vi "ParamByteArray.vi"(2 "idx":u8, 3 "Param Nm":u8) -> (5 "Byte3":u8, 6 "Byte2":u8, 7 "Byte1":u8, 8 "Byte0":u8)   [LabVIEW 2017]
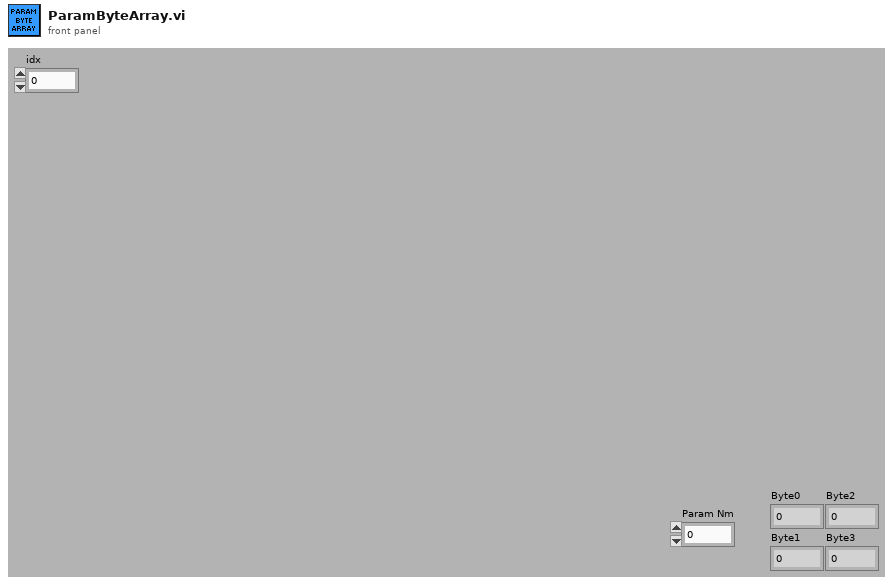
[diagram p1: front panel]
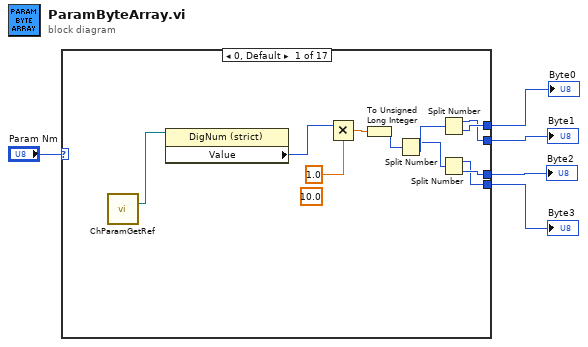
[diagram p0: block diagram]
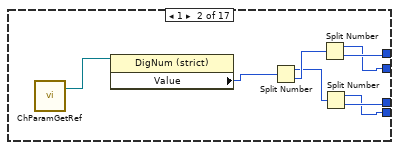
[diagram p2: hidden frame]
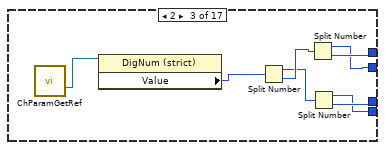
[diagram p3: hidden frame]
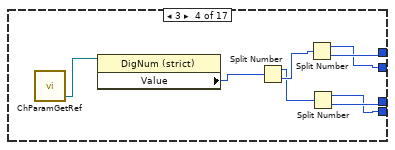
[diagram p4: hidden frame]
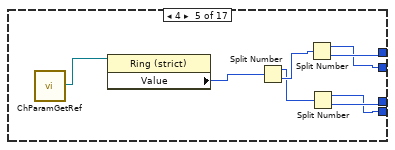
[diagram p5: hidden frame]
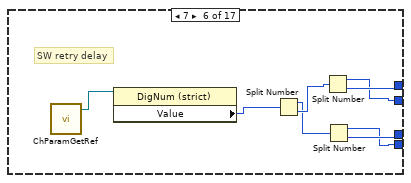
[diagram p6: hidden frame]
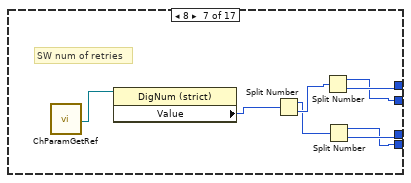
[diagram p7: hidden frame]
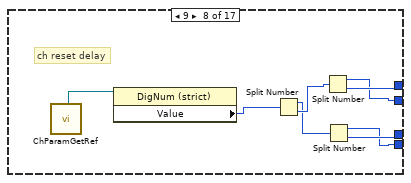
[diagram p8: hidden frame]
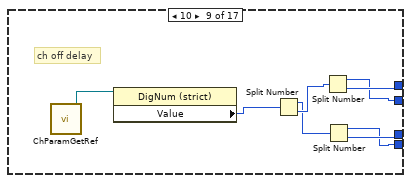
[diagram p9: hidden frame]
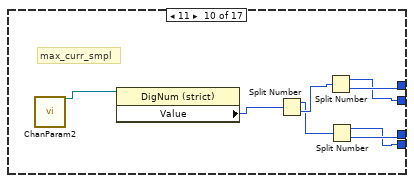
[diagram p10: hidden frame]
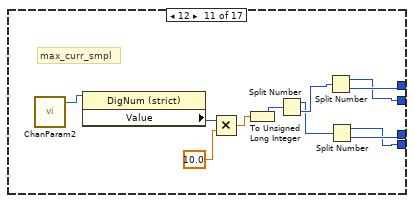
[diagram p11: hidden frame]
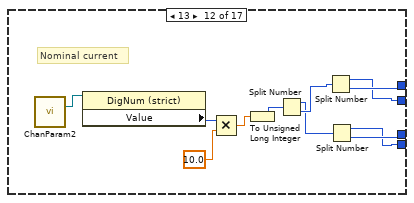
[diagram p12: hidden frame]
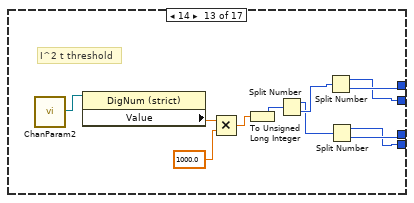
[diagram p13: hidden frame]
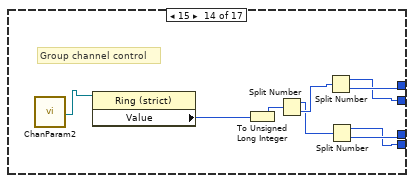
[diagram p14: hidden frame]
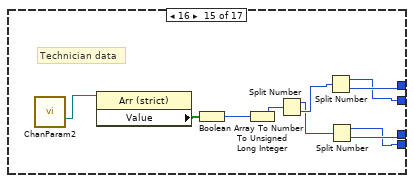
[diagram p15: hidden frame]
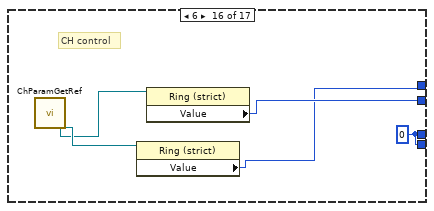
[diagram p16: hidden frame]
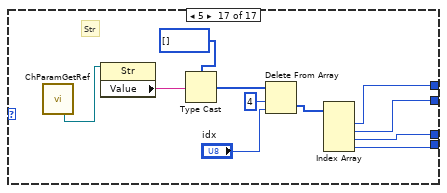
[diagram p17: hidden frame]
diagram:
  n1 = case shown="0, Default" "Param Nm" {
    tunnel: [w14 w20 w28 w36 w45 w53 w61 w69 w77 w85 w97 w108 w119 w128 w138 w142 w150] -> w4
    tunnel: [w13 w19 w27 w35 w44 w52 w60 w68 w76 w84 w96 w107 w118 w127 w137 w143 w149] -> w3
    tunnel: [w12 w18 w26 w34 w43 w51 w59 w67 w75 w83 w95 w106 w117 w126 w136 w141 w148] -> w2
    tunnel: [w11 w17 w25 w33 w42 w50 w58 w66 w74 w82 w94 w105 w116 w125 w135 w141 w147] -> w1
    frame 0, Default {
      (unwired) 10.0 ("y")
      n2 = call "ChParamGetRef.vi"() -> ("Current Threshold  out"=w6:refnum<vi>)  [unwired: 15 in, 12 out]
      n3 = property class="DigNum (strict)"(reference=w6) -> ("Value"=w7:u32)  [unwired: 1 in, 2 out]
      n4 = Multiply(x=w7, y=1.0) -> (x*y=w10:dbl)
      n5 = To Unsigned Long Integer(number=w10) -> (unsigned 32bit integer=w9:u32)
      n6 = Split Number(x=w9) -> (hi(x)=w15:u16, lo(x)=w16:u16)
      n7 = Split Number(x=w16) -> (hi(x)=w13:u8, lo(x)=w14:u8)
      n8 = Split Number(x=w15) -> (hi(x)=w11:u8, lo(x)=w12:u8)
    }
    frame 1 {
      n9 = call "ChParamGetRef.vi"() -> ("Channel On Delay out"=w23:refnum<vi>)  [unwired: 15 in, 12 out]
      n10 = property class="DigNum (strict)"(reference=w23) -> ("Value"=w24:u32)  [unwired: 1 in, 2 out]
      n11 = Split Number(x=w24) -> (hi(x)=w21:u16, lo(x)=w22:u16)
      n12 = Split Number(x=w22) -> (hi(x)=w19:u8, lo(x)=w20:u8)
      n13 = Split Number(x=w21) -> (hi(x)=w17:u8, lo(x)=w18:u8)
    }
    frame 2 {
      n14 = call "ChParamGetRef.vi"() -> ("Retry Delay out"=w31:refnum<vi>)  [unwired: 15 in, 12 out]
      n15 = property class="DigNum (strict)"(reference=w31) -> ("Value"=w32:u32)  [unwired: 1 in, 2 out]
      n16 = Split Number(x=w32) -> (hi(x)=w29:u16, lo(x)=w30:u16)
      n17 = Split Number(x=w30) -> (hi(x)=w27:u8, lo(x)=w28:u8)
      n18 = Split Number(x=w29) -> (hi(x)=w25:u8, lo(x)=w26:u8)
    }
    frame 3 {
      n19 = call "ChParamGetRef.vi"() -> ("Number Of Retry out"=w39:refnum<vi>)  [unwired: 15 in, 12 out]
      n20 = property class="DigNum (strict)"(reference=w39) -> ("Value"=w40:u32)  [unwired: 1 in, 2 out]
      n21 = Split Number(x=w40) -> (hi(x)=w37:u16, lo(x)=w38:u16)
      n22 = Split Number(x=w38) -> (hi(x)=w35:u8, lo(x)=w36:u8)
      n23 = Split Number(x=w37) -> (hi(x)=w33:u8, lo(x)=w34:u8)
    }
    frame 4 {
      n24 = call "ChParamGetRef.vi"() -> ("Active on startup out"=w41:refnum<vi>)  [unwired: 15 in, 12 out]
      n25 = property class="Ring (strict)"(reference=w41) -> ("Value"=w48:u8)  [unwired: 1 in, 2 out]
      n26 = Split Number(x=w48) -> (hi(x)=w46:u8, lo(x)=w47:u8)
      n27 = Split Number(x=w47) -> (hi(x)=w44:u8, lo(x)=w45:u8)
      n28 = Split Number(x=w46) -> (hi(x)=w42:u8, lo(x)=w43:u8)
    }
    frame 7 {
      # "SW retry delay"
      n29 = call "ChParamGetRef.vi"() -> ("SW Retry Delay out"=w49:refnum<vi>)  [unwired: 15 in, 12 out]
      n30 = property class="DigNum (strict)"(reference=w49) -> ("Value"=w56:u32)  [unwired: 1 in, 2 out]
      n31 = Split Number(x=w56) -> (hi(x)=w54:u16, lo(x)=w55:u16)
      n32 = Split Number(x=w55) -> (hi(x)=w52:u8, lo(x)=w53:u8)
      n33 = Split Number(x=w54) -> (hi(x)=w50:u8, lo(x)=w51:u8)
    }
    frame 8 {
      # "SW num of retries"
      n34 = call "ChParamGetRef.vi"() -> ("SW Number Of Retry out"=w57:refnum<vi>)  [unwired: 15 in, 12 out]
      n35 = property class="DigNum (strict)"(reference=w57) -> ("Value"=w64:u32)  [unwired: 1 in, 2 out]
      n36 = Split Number(x=w64) -> (hi(x)=w62:u16, lo(x)=w63:u16)
      n37 = Split Number(x=w63) -> (hi(x)=w60:u8, lo(x)=w61:u8)
      n38 = Split Number(x=w62) -> (hi(x)=w58:u8, lo(x)=w59:u8)
    }
    frame 9 {
      # "ch reset delay"
      n39 = call "ChParamGetRef.vi"() -> ("Reset Status Delay out"=w65:refnum<vi>)  [unwired: 15 in, 12 out]
      n40 = property class="DigNum (strict)"(reference=w65) -> ("Value"=w72:u32)  [unwired: 1 in, 2 out]
      n41 = Split Number(x=w72) -> (hi(x)=w70:u16, lo(x)=w71:u16)
      n42 = Split Number(x=w71) -> (hi(x)=w68:u8, lo(x)=w69:u8)
      n43 = Split Number(x=w70) -> (hi(x)=w66:u8, lo(x)=w67:u8)
    }
    frame 10 {
      # "ch off delay"
      n44 = call "ChParamGetRef.vi"() -> ("Channel OFF delay out"=w73:refnum<vi>)  [unwired: 15 in, 12 out]
      n45 = property class="DigNum (strict)"(reference=w73) -> ("Value"=w80:u32)  [unwired: 1 in, 2 out]
      n46 = Split Number(x=w80) -> (hi(x)=w78:u16, lo(x)=w79:u16)
      n47 = Split Number(x=w79) -> (hi(x)=w76:u8, lo(x)=w77:u8)
      n48 = Split Number(x=w78) -> (hi(x)=w74:u8, lo(x)=w75:u8)
    }
    frame 11 {
      # "max_curr_smpl"
      n49 = call "ChanParam2.vi"() -> ("Num.MaxCurrTime out"=w81:refnum<vi>)  [unwired: 22 in, 5 out]
      n50 = property class="DigNum (strict)"(reference=w81) -> ("Value"=w88:u32)  [unwired: 1 in, 2 out]
      n51 = Split Number(x=w88) -> (hi(x)=w86:u16, lo(x)=w87:u16)
      n52 = Split Number(x=w87) -> (hi(x)=w84:u8, lo(x)=w85:u8)
      n53 = Split Number(x=w86) -> (hi(x)=w82:u8, lo(x)=w83:u8)
    }
    frame 12 {
      # "max_curr_smpl"
      n54 = call "ChanParam2.vi"() -> ("I Max Threshold out"=w93:refnum<vi>)  [unwired: 22 in, 5 out]
      n55 = property class="DigNum (strict)"(reference=w93) -> ("Value"=w90:u32)  [unwired: 1 in, 2 out]
      n56 = Multiply(x=w90, y=10.0) -> (x*y=w92:dbl)
      n57 = To Unsigned Long Integer(number=w92) -> (unsigned 32bit integer=w89:u32)
      n58 = Split Number(x=w89) -> (hi(x)=w98:u16, lo(x)=w99:u16)
      n59 = Split Number(x=w99) -> (hi(x)=w96:u8, lo(x)=w97:u8)
      n60 = Split Number(x=w98) -> (hi(x)=w94:u8, lo(x)=w95:u8)
    }
    frame 13 {
      # "Nominal current"
      n61 = call "ChanParam2.vi"() -> ("I Nominal out"=w100:refnum<vi>)  [unwired: 22 in, 5 out]
      n62 = property class="DigNum (strict)"(reference=w100) -> ("Value"=w102:u32)  [unwired: 1 in, 2 out]
      n63 = Multiply(x=w102, y=10.0) -> (x*y=w104:dbl)
      n64 = To Unsigned Long Integer(number=w104) -> (unsigned 32bit integer=w101:u32)
      n65 = Split Number(x=w101) -> (hi(x)=w109:u16, lo(x)=w110:u16)
      n66 = Split Number(x=w110) -> (hi(x)=w107:u8, lo(x)=w108:u8)
      n67 = Split Number(x=w109) -> (hi(x)=w105:u8, lo(x)=w106:u8)
    }
    frame 14 {
      # "I^2 t threshold"
      n68 = call "ChanParam2.vi"() -> ("I2t out"=w111:refnum<vi>)  [unwired: 22 in, 5 out]
      n69 = property class="DigNum (strict)"(reference=w111) -> ("Value"=w113:dbl)  [unwired: 1 in, 2 out]
      n70 = Multiply(x=w113, y=1000.0) -> (x*y=w115:dbl)
      n71 = To Unsigned Long Integer(number=w115) -> (unsigned 32bit integer=w112:u32)
      n72 = Split Number(x=w112) -> (hi(x)=w120:u16, lo(x)=w121:u16)
      n73 = Split Number(x=w121) -> (hi(x)=w118:u8, lo(x)=w119:u8)
      n74 = Split Number(x=w120) -> (hi(x)=w116:u8, lo(x)=w117:u8)
    }
    frame 15 {
      # "Group channel control"
      n75 = call "ChanParam2.vi"() -> ("Group control out"=w123:refnum<vi>)  [unwired: 22 in, 5 out]
      n76 = property class="Ring (strict)"(reference=w123) -> ("Value"=w122:u8)  [unwired: 1 in, 2 out]
      n77 = To Unsigned Long Integer(number=w122) -> (unsigned 32bit integer=w124:u32)
      n78 = Split Number(x=w124) -> (hi(x)=w129:u16, lo(x)=w130:u16)
      n79 = Split Number(x=w130) -> (hi(x)=w127:u8, lo(x)=w128:u8)
      n80 = Split Number(x=w129) -> (hi(x)=w125:u8, lo(x)=w126:u8)
    }
    frame 16 {
      # "Technician data"
      n81 = call "ChanParam2.vi"() -> ("Tech.Data out"=w133:refnum<vi>)  [unwired: 22 in, 5 out]
      n82 = property class="Arr (strict)"(reference=w133) -> ("Value"=w132:bool[])  [unwired: 1 in, 2 out]
      n83 = Boolean Array To Number(Boolean array=w132) -> (number=w131:u32)
      n84 = To Unsigned Long Integer(number=w131) -> (unsigned 32bit integer=w134:u32)
      n85 = Split Number(x=w134) -> (hi(x)=w139:u16, lo(x)=w140:u16)
      n86 = Split Number(x=w140) -> (hi(x)=w137:u8, lo(x)=w138:u8)
      n87 = Split Number(x=w139) -> (hi(x)=w135:u8, lo(x)=w136:u8)
    }
    frame 6 {
      w141 = u8 0
      # "CH control"
      n88 = call "ChParamGetRef.vi"() -> ("Comm. control out"=w144:refnum<vi>, "I/O control out"=w145:refnum<vi>)  [unwired: 15 in, 11 out]
      n89 = property class="Ring (strict)"(reference=w145) -> ("Value"=w142:u8)  [unwired: 1 in, 2 out]
      n90 = property class="Ring (strict)"(reference=w144) -> ("Value"=w143:u8)  [unwired: 1 in, 2 out]
    }
    frame 5 {
      # "Str"
      n91 = call "ChParamGetRef.vi"() -> ("Ch General data out"=w146:refnum<vi>)  [unwired: 15 in, 12 out]
      n92 = property class="Str"(reference=w146) -> ("Value"=w156:string)  [unwired: 1 in, 2 out]
      n93 = Type Cast(type=u8[] [], x=w156) -> (*(type *) &x=w154:u8[])
      n94 = Delete From Array(array=w154, length=4, index="idx") -> (deleted portion=w151:u8[])  [unwired: 1 out]
      n95 = Index Array(array=w151) -> (element #1=w150:u8, element #2=w149:u8, element #3=w148:u8, element #4=w147:u8)  [unwired: 4 in]
    }
  }
  "Byte0" <- w4
  "Byte1" <- w3
  "Byte2" <- w2
  "Byte3" <- w1
